vi "Constructor_LogHandle.vi"(7 "Formatter":refnum<class "ILogFormatter.lvclass">, 8 "error in (no error)":errorcluster, 10 "INetworkWriter":refnum<class "INetworkWriter.lvclass">) -> (0 "error out":errorcluster, 3 "FileHandler out":refnum<class "StreamLogHandle.lvclass">)   [LabVIEW 2024, in "StreamLogHandle.lvclass"]
uses:
  StreamLogHandle.lvclass
  Stream/INetworkWriter/INetworkWriter.lvclass
  LogFormatter/Interface/ILogFormatter.lvclass
  StreamLogHandle.lvclass/StreamLogHandle.ctl
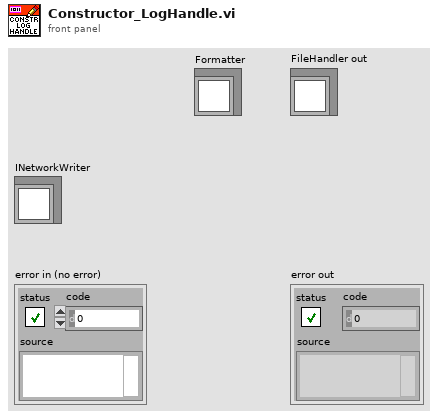
[diagram p1: front panel]
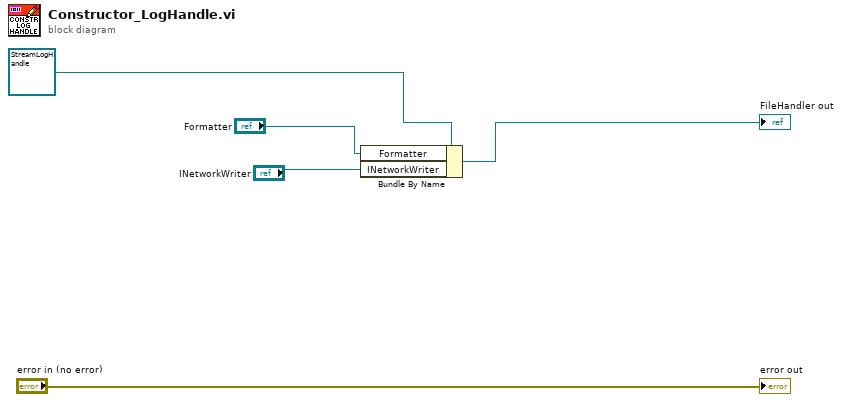
[diagram p0: block diagram]
diagram:
  n1 = Bundle By Name(cluster=refnum<class "StreamLogHandle.lvclass"> refnum ("FileHandler in"), "Formatter"="Formatter", "INetworkWriter"="INetworkWriter") -> (→"FileHandler out":refnum<class "StreamLogHandle.lvclass">)
  "error out" <- "error in (no error)"
